vi "Reorder Tasks.vi"(10 "Indices":i32[](array[numeric]), 11 "Tasks in":refnum<k21>[](array[refnum])) -> (3 "Tasks out":refnum<k21>[](array[refnum]))   [LabVIEW 2019, in "Instrument.DAQ.lvclass"]
uses:
  Instrument.DAQ.lvclass
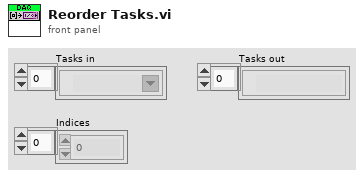
[diagram p1: front panel]
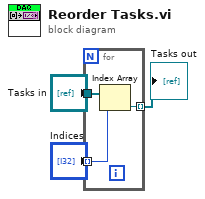
[diagram p0: block diagram]
diagram:
  n1 = for {
    tunnel: "Indices" -> [w4] mode=indexing
    tunnel: "Tasks in" -> [w6]
    tunnel: [w5] -> w3 mode=indexing
    n2 = Index Array(array=w6, index=w4) -> (element=w5:refnum<k21>)
  }
  "Tasks out" <- w3
